vi "clear keys.vi"(8 "error in":errorcluster, 11 "lvlibretls configurable context in":refnum<class "lvlibretls configurable context.lvclass">) -> (0 "error out":errorcluster, 3 "lvlibretls configurable context out":refnum<class "lvlibretls configurable context.lvclass">)   [LabVIEW 2016, in "lvlibretls configurable context.lvclass"]
uses:
  lvlibretls configurable context.lvclass
  lvlibretls configurable context.lvclass/lvlibretls configurable context.ctl
  lv tls dll.lvlib
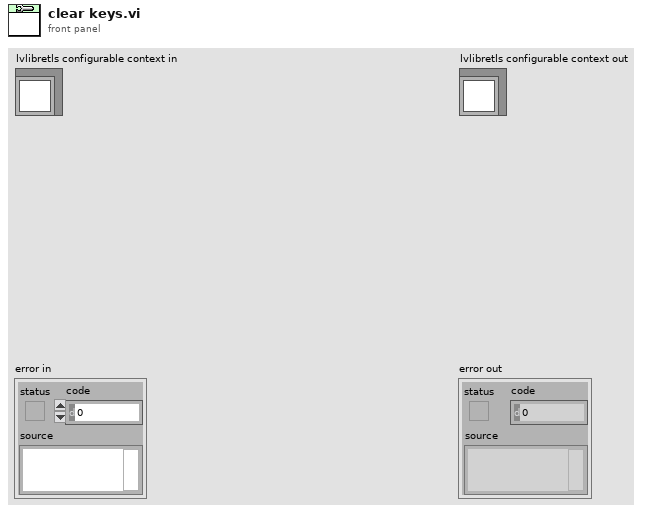
[diagram p1: front panel]
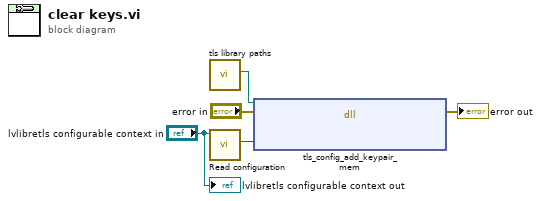
[diagram p0: block diagram]
diagram:
  n1 = call "tls library paths.vi"() -> ("libtls"=w5:path)  [unwired: 8 in, 3 out]
  n2 = call "Read configuration.vi"("lvlibretls configurable context in"="lvlibretls configurable context in") -> ("configuration"=w4:u64)  [unwired: 10 in]
  n3 = dll-call lib="C:/Users/IEUser/Desktop/tlssimple/libtls-15.dll" fn="tls_config_add_keypair_mem"(path in=w5, error in="error in", "config"=w4) -> (error out=→"error out":errorcluster)  [unwired: 3 in, 1 out]
  "lvlibretls configurable context out" <- "lvlibretls configurable context in"
